vi "Configure Limit Line Edit.vi"(0 "VISA resource name":refnum<visa-resource-name>, 5 "Limit Line (1)":i32=1 min=1 max=6, 7 "Line Setting":T1(array[cluster]), 11 "error in (no error)":errorcluster) -> (4 "VISA resource name out":refnum<visa-resource-name>, 15 "error out":errorcluster)   [LabVIEW 2020, in "Anritsu Signal Analyzer Series.lvlib"]
doc: "Configures the Frequency, Amplitude, and Connected to Previous Pt parameters for Limit Points on the specified Limit Line."
uses:
  Anritsu Signal Analyzer Series.lvlib
panel:
  # "Hz"
  # "dB"
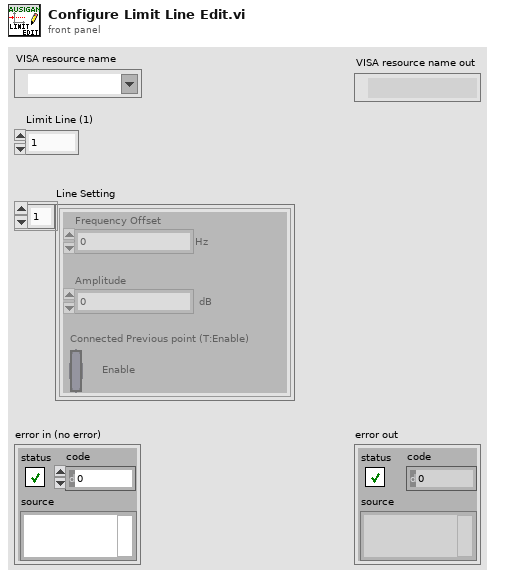
[diagram p1: front panel]
types:
  T1 = cluster{"Frequency Offset ":dbl, "Amplitude":dbl, "Connected Previous point (T:Enable)":bool}[]
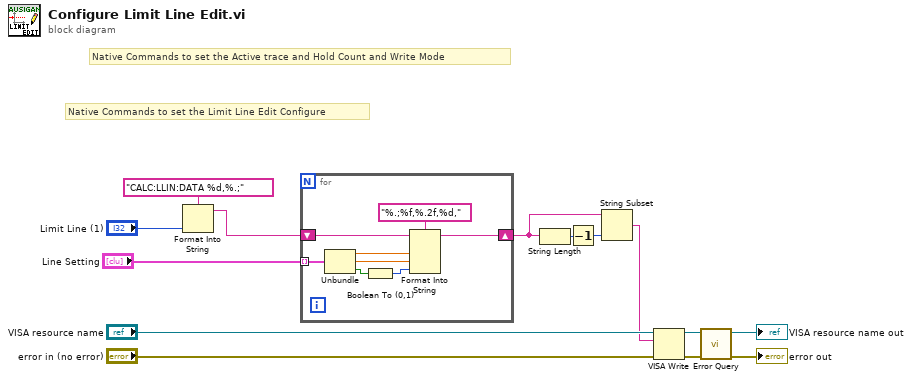
[diagram p0: block diagram]
diagram:
  # "Native Commands to set the Limit Line Edit Configure"
  # "Native Commands to set the Active trace and Hold Count and Write Mode"
  n1 = Format Into String(format string="CALC:LLIN:DATA %d,%.;", "Limit Line (1)") -> (resulting string=w5:string)  [unwired: 2 in, 1 out]
  n2 = for {
    tunnel: "Line Setting" -> [w21] mode=indexing
    shift-right: [w15] -> w2
    shift-left: w5 -> [w16]
    n3 = Unbundle(w21) -> ("Frequency Offset"=w20:dbl, "Amplitude"=w19:dbl, "Connected Previous point (T:Enable)"=w18:bool)
    n4 = Boolean To (0,1)(Boolean=w18) -> (0, 1=w17:i16)
    n5 = Format Into String(format string="%.;%f,%.2f,%d,", initial string=w16, w20, w19, w17) -> (resulting string=w15:string)  [unwired: 1 in, 1 out]
  }
  n6 = String Length(string=w2) -> (length=w4:i32)
  n7 = Decrement(x=w4) -> (x-1=w3:i32)
  n8 = String Subset(string=w2, length (rest)=w3) -> (substring=w1:string)  [unwired: 1 in]
  n9 = VISA Write(VISA resource name="VISA resource name", write buffer=w1, error in (no error)="error in (no error)") -> (VISA resource name out=w10:refnum<visa-resource-name>, error out=w9:errorcluster)  [unwired: 1 out]
  n10 = call "Error Query.vi"("error in (no error)"=w9, "VISA resource name"=w10) -> ("error out"=→"error out":errorcluster, "VISA resource name out"=→"VISA resource name out":refnum<visa-resource-name>)  [unwired: 6 in, 2 out]
